vi "Create Coverage Analyzer View.vi"(8 "error in (no error)":errorcluster, 11 "Coverage Analyzer Result View in":T1) -> (0 "error out":errorcluster, 3 "Coverage Analyzer Result View out":refnum<class "Coverage Analyzer Result View.lvclass">)   [LabVIEW 2020, in "Coverage Analyzer Result View.lvclass"]
uses:
  Coverage Analyzer Result View.lvclass
  Coverage Analyzer View Data.ctl
  Coverage Analyzer Result View.lvclass/Coverage Analyzer Result View.ctl
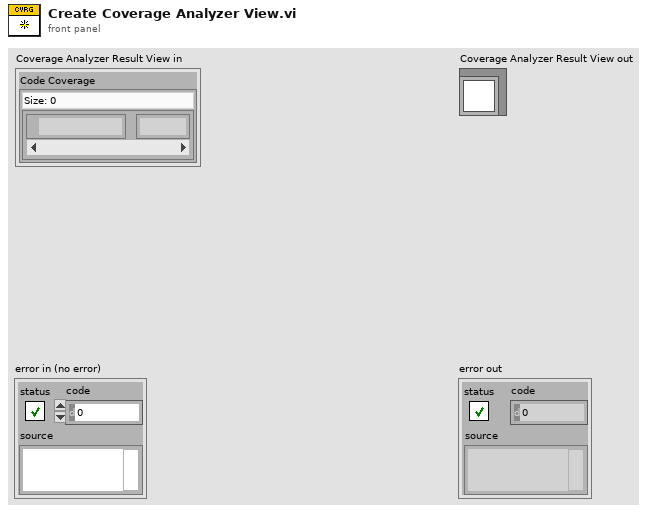
[diagram p1: front panel]
types:
  T1 = typedef "Coverage Analyzer Result View.lvclass/Coverage Analyzer View Data.ctl" = cluster{"Code Coverage":map{path, dbl}}
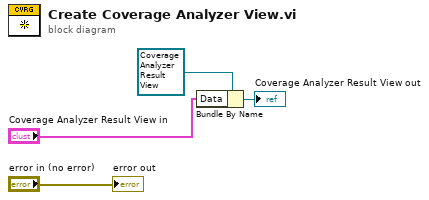
[diagram p0: block diagram]
diagram:
  n1 = Bundle By Name(cluster=refnum<class "Coverage Analyzer Result View.lvclass"> refnum ("Coverage Analyzer Result View.lvclass"), "Data"="Coverage Analyzer Result View in") -> (→"Coverage Analyzer Result View out":refnum<class "Coverage Analyzer Result View.lvclass">)
  "error out" <- "error in (no error)"
